vi "Encode.vi"(8 "error in (no error)":errorcluster, 10 "Data":i16[](array[numeric]), 11 "Actuator in":refnum<class "Actuator.lvclass">) -> (0 "error out":errorcluster, 2 "Message":string, 3 "Actuator out":refnum<class "Actuator.lvclass">)   [LabVIEW 2021, in "Actuator.lvclass"]
uses:
  Actuator.lvclass
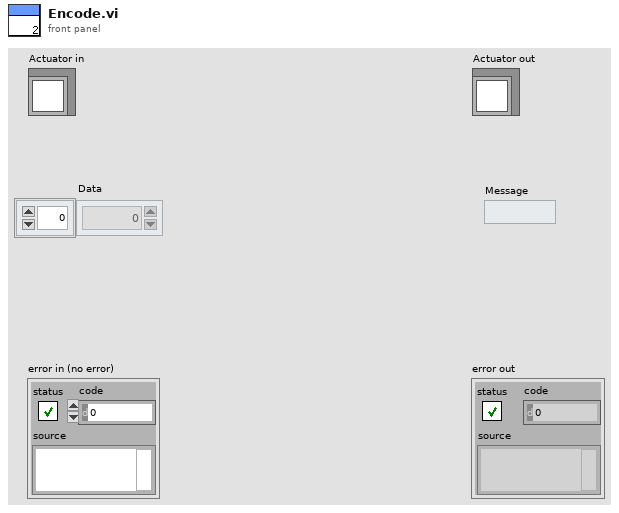
[diagram p1: front panel]
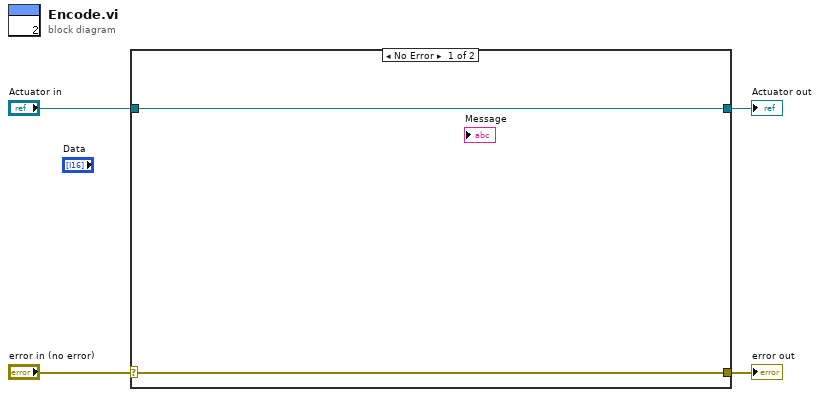
[diagram p0: block diagram]
diagram:
  n1 = case shown="No Error" "error in (no error)" {
    selector: "error in (no error)" -> [w5 w8]
    tunnel: [w5 w8] -> w3
    tunnel: [w6 w7] -> w1
    tunnel: "Actuator in" -> [w6 w7]
    frame No Error {
    }
    frame Error {
    }
  }
  "error out" <- w3
  "Actuator out" <- w1
